vi "auto gripper.vi"(9 "button 9":bool, 10 "button 2":bool, 11 "encoder distance":dbl) -> (2 "change state":bool, 3 "gripper state":bool)   [LabVIEW 2011]
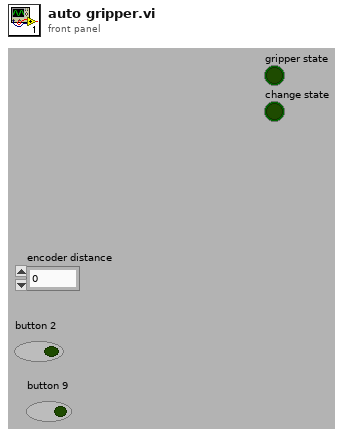
[diagram p1: front panel]
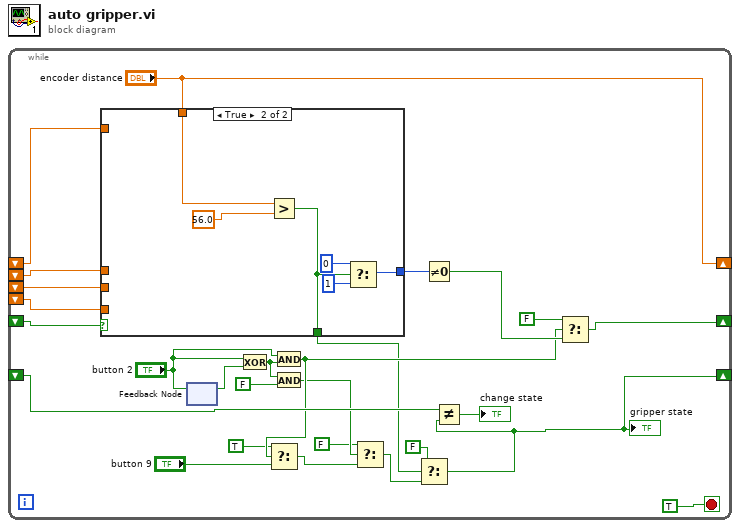
[diagram p0: block diagram]
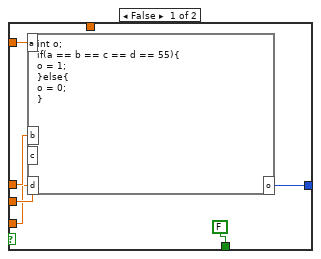
[diagram p2: hidden frame]
diagram:
  n1 = while {
    shift-right: ["encoder distance"] -> _
    shift-left: _ -> [w26]
    shift-left: _ -> [w25]
    shift-left: _ -> [w24]
    shift-left: _ -> [w23]
    shift-right: [w16] -> _
    shift-left: _ -> [w21]
    shift-right: [w1] -> _
    shift-left: _ -> [w15]
    stop <- TRUE stop-if-true
    n2 = case shown="True" w21 {
      tunnel: w26 -> [w33 _]
      tunnel: w25 -> [w32 _]
      tunnel: w24 -> [w31 _]
      tunnel: w23 -> [w30 _]
      tunnel: [w29 w37] -> w22
      tunnel: "encoder distance" -> [_ w38]
      tunnel: [FALSE w34] -> w8
      frame False {
        n3 = formula code="int o;\nif(a == b == c == d == 55){\no = 1;\n}else{\no = 0;\n}"("a"=w33, "b"=w32, "c"=w31, "d"=w30) -> ("o"=w29:i32)
      }
      frame True {
        n4 = Greater?(x=w38, y=56.0) -> (0:w34:bool)
        n5 = Select(t=0, s=w34, f=1) -> (s? t:f=w37:i32)
      }
    }
    n6 = feedback-in #1("button 2") -> ()
    n7 = feedback #1() -> (w19:bool)  [unwired: 1 out]
    n8 = Exclusive Or(1:w19, 2:"button 2") -> (0:w11:bool)
    n9 = And(x="button 2", y=w11) -> (x .and. y?=w12:bool)
    n10 = Select(t=TRUE, s=w12, f="button 9") -> (s? t:f=w5:bool)
    n11 = And(x=w11, y=FALSE) -> (x .and. y?=w9:bool)
    n12 = Select(t=FALSE, s=w9, f=w5) -> (s? t:f=w3:bool)
    n13 = Select(t=FALSE, s=w8, f=w3) -> (s? t:f=w1:bool)
    "gripper state" <- w1
    n14 = Not Equal To 0?(x=w22) -> (x != 0?=w18:bool)
    n15 = Not Equal?(x=w15, y=w1) -> (x != y?=→"change state":bool)
    n16 = Select(t=FALSE, s=w12, f=w18) -> (s? t:f=w16:bool)
  }
